vi "TCPClient.vi"() -> ()   [LabVIEW 2020]
uses:
  <vilib>/Analysis/4window.llb/Hanning Window (DBL).vi
  <vilib>/Analysis/4window.llb/AllCosWindow (DBL).vi
  <vilib>/Analysis/NI_AALPro.lvlib
  <vilib>/Analysis/NI_AALBase.lvlib
panel:
  in  "right rank 3":i32=-1
  in  "left rank 3":i32=2
  out "?":i32
  out "max value":i32
  out "Виброускорение":dbl[](graph)
  in  "right rank 2":i32=-1
  in  "left rank 2":i32=2
  in  "right rank":i32=-1
  in  "left rank":i32=2
  out "Виброскорость":dbl[](graph)
  out "Индекс А":i32
  out "Индекс":i32
  out "Максимальная амплитуда на спектре A":dbl
  out "Максимальная амплитуда на спектре S":dbl
  out "error out":errorcluster
  out "Спектр виброускорение":dbl[](graph)
  out "df 2":dbl
  out "СКЗ виброускорения":dbl
  out "Спектр виброскорость":dbl[](graph)
  out "df":dbl
  out "СКЗ Виброскорости":dbl
  out "Виброперемещение":i32[][](graph)
  in  "Connection Uuid":string
  in  "local port (0)":u16
  in  "address 127.0.0.1":string
  # "Панель подключения"
  # "Амплитуда"
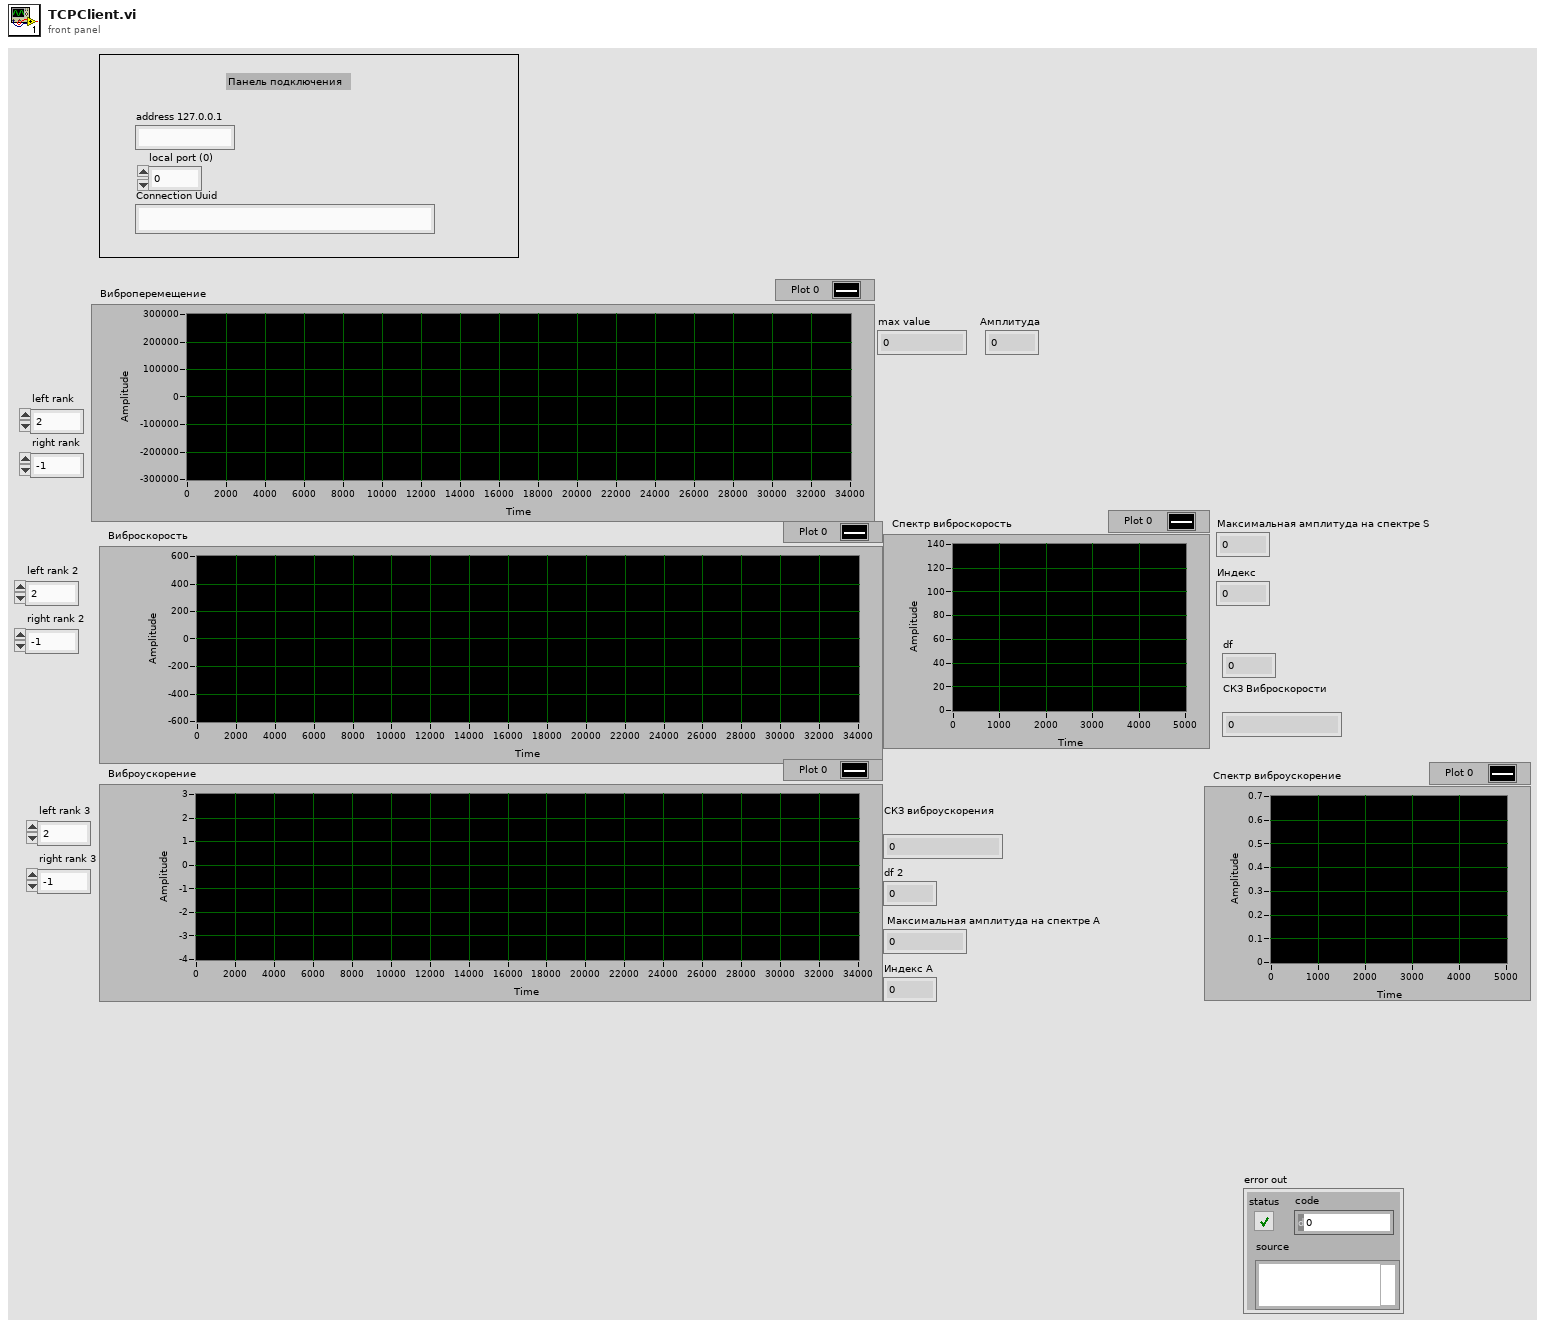
[diagram p1: front panel]
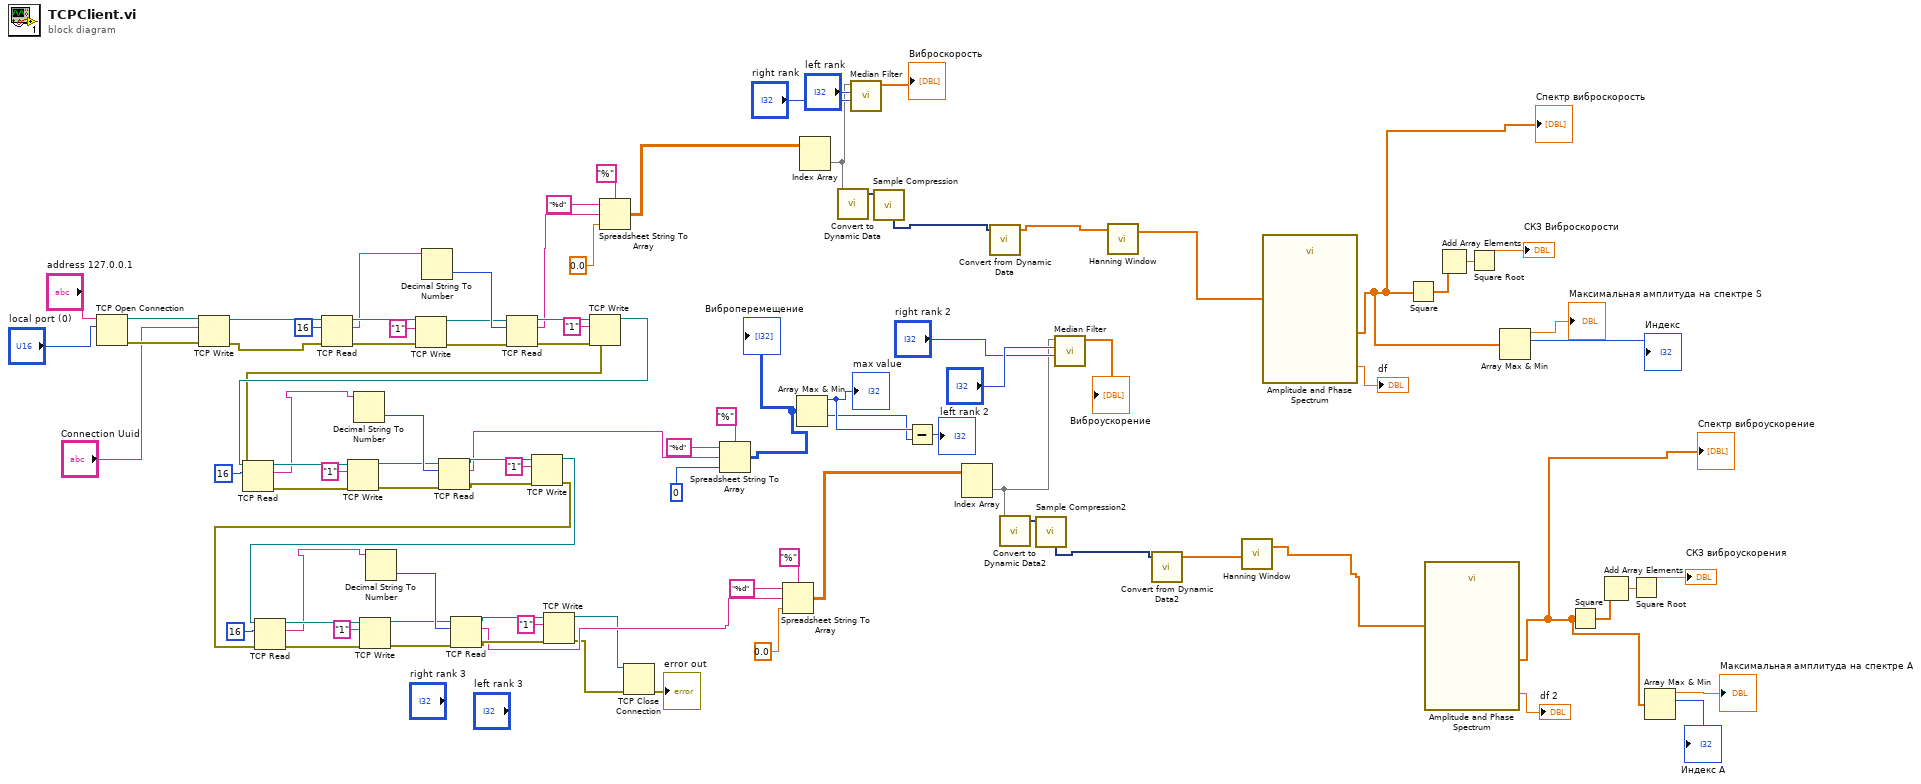
[diagram p0: block diagram]
diagram:
  n1 = TCP Open Connection(address="address 127.0.0.1", remote port or service name="local port (0)") -> (connection ID=w95:refnum<k5>, error out=w94:errorcluster)  [unwired: 3 in]
  n2 = TCP Write(connection ID=w95, data in="Connection Uuid", error in (no error)=w94) -> (connection ID out=w90:refnum<k5>, error out=w91:errorcluster)  [unwired: 1 in, 1 out]
  n3 = TCP Read(connection ID=w90, bytes to read=16, error in (no error)=w91) -> (connection ID out=w87:refnum<k5>, data out=w85:string, error out=w88:errorcluster)  [unwired: 2 in]
  n4 = TCP Write(connection ID=w87, data in="1", error in (no error)=w88) -> (connection ID out=w83:refnum<k5>, error out=w82:errorcluster)  [unwired: 1 in, 1 out]
  n5 = Decimal String To Number(string=w85) -> (number=w84:i32)  [unwired: 2 in, 1 out]
  n6 = TCP Read(connection ID=w83, bytes to read=w84, error in (no error)=w82) -> (connection ID out=w80:refnum<k5>, data out=w17:string, error out=w79:errorcluster)  [unwired: 2 in]
  n7 = TCP Write(connection ID=w80, data in="1", error in (no error)=w79) -> (connection ID out=w53:refnum<k5>, error out=w52:errorcluster)  [unwired: 1 in, 1 out]
  n8 = TCP Read(connection ID=w53, bytes to read=16, error in (no error)=w52) -> (connection ID out=w73:refnum<k5>, data out=w68:string, error out=w74:errorcluster)  [unwired: 2 in]
  n9 = TCP Write(connection ID=w73, data in="1", error in (no error)=w74) -> (connection ID out=w70:refnum<k5>, error out=w69:errorcluster)  [unwired: 1 in, 1 out]
  n10 = Decimal String To Number(string=w68) -> (number=w71:i32)  [unwired: 2 in, 1 out]
  n11 = TCP Read(connection ID=w70, bytes to read=w71, error in (no error)=w69) -> (connection ID out=w65:refnum<k5>, data out=w46:string, error out=w66:errorcluster)  [unwired: 2 in]
  n12 = TCP Write(connection ID=w65, data in="1", error in (no error)=w66) -> (connection ID out=w50:refnum<k5>, error out=w51:errorcluster)  [unwired: 1 in, 1 out]
  n13 = TCP Read(connection ID=w50, bytes to read=16, error in (no error)=w51) -> (connection ID out=w62:refnum<k5>, data out=w57:string, error out=w63:errorcluster)  [unwired: 2 in]
  n14 = TCP Write(connection ID=w62, data in="1", error in (no error)=w63) -> (connection ID out=w59:refnum<k5>, error out=w58:errorcluster)  [unwired: 1 in, 1 out]
  n15 = Decimal String To Number(string=w57) -> (number=w60:i32)  [unwired: 2 in, 1 out]
  n16 = TCP Read(connection ID=w59, bytes to read=w60, error in (no error)=w58) -> (connection ID out=w54:refnum<k5>, data out=w43:string, error out=w55:errorcluster)  [unwired: 2 in]
  n17 = TCP Write(connection ID=w54, data in="1", error in (no error)=w55) -> (connection ID out=w30:refnum<k5>, error out=w29:errorcluster)  [unwired: 1 in, 1 out]
  n18 = Spreadsheet String To Array(delimiter (Tab)="%", format string="%d", spreadsheet string=w17, array type (2D Dbl)=0.0) -> (array=w13:dbl[][])
  n19 = TCP Close Connection(connection ID=w30, error in (no error)=w29) -> (error out=→"error out":errorcluster)  [unwired: 1 in, 1 out]
  n20 = Spreadsheet String To Array(delimiter (Tab)="%", format string="%d", spreadsheet string=w46, array type (2D Dbl)=0) -> (array=w2:i32[][])
  "Виброперемещение" <- w2
  n21 = Spreadsheet String To Array(delimiter (Tab)="%", format string="%d", spreadsheet string=w43, array type (2D Dbl)=0.0) -> (array=w15:dbl[][])
  n22 = Array Max & Min(array=w2) -> (max value=w5:i32, min value=w4:i32)  [unwired: 2 out]
  "max value" <- w5
  n23 = Index Array(array=w13) -> (element=w1:dbl[])  [unwired: 2 in]
  n24 = call "Convert to Dynamic Data"("Array"=w1) -> ("Dynamic Data Type"=w38:dynamicdata)  [unwired: 3 in]
  n25 = call <vilib>:"Median Filter.vi"("right rank"="right rank", "left rank"="left rank", "X"=w1) -> ("Filtered X"=→"Виброскорость":dbl[])  [unwired: 7 in, 1 out]
  n26 = call "Sample Compression"("Signals"=w38) -> ("Last"=w27:dynamicdata)  [unwired: 8 in, 2 out]
  n27 = Subtract(x=w5, y=w4) -> (x-y=→"?":i32)
  n28 = Index Array(array=w15) -> (element=w7:dbl[])  [unwired: 2 in]
  n29 = call "Convert from Dynamic Data"("Dynamic Data Type"=w27) -> ("Array"=w24:dbl[])  [unwired: 3 in]
  n30 = call "Convert to Dynamic Data2"("Array"=w7) -> ("Dynamic Data Type"=w33:dynamicdata)  [unwired: 3 in]
  n31 = call "Sample Compression2"("Signals"=w33) -> ("Last"=w26:dynamicdata)  [unwired: 8 in, 2 out]
  n32 = call <vilib>:"Median Filter.vi"("right rank"="right rank 2", "left rank"="left rank 2", "X"=w7) -> ("Filtered X"=→"Виброускорение":dbl[])  [unwired: 7 in, 1 out]
  n33 = call-poly <vilib>:"Hanning Window.vi"("X"=w24) -> ("Windowed X"=w14:dbl[])  [unwired: 1 out]
  n34 = call "Convert from Dynamic Data2"("Dynamic Data Type"=w26) -> ("Array"=w25:dbl[])  [unwired: 3 in]
  n35 = call-poly <vilib>:"Hanning Window.vi"("X"=w25) -> ("Windowed X"=w16:dbl[])  [unwired: 1 out]
  n36 = call <vilib>:"Amplitude and Phase Spectrum.vi"("Signal (V)"=w14) -> ("df"=→"df":dbl, "Amp Spectrum Mag (Vrms)"=w23:dbl[])  [unwired: 2 in, 1 out]
  "Спектр виброскорость" <- w23
  n37 = Square(x=w23) -> (x^2=w41:dbl[])
  n38 = call <vilib>:"Amplitude and Phase Spectrum.vi"("Signal (V)"=w16) -> ("df"=→"df 2":dbl, "Amp Spectrum Mag (Vrms)"=w21:dbl[])  [unwired: 2 in, 1 out]
  "Спектр виброускорение" <- w21
  n39 = Add Array Elements(numeric array=w41) -> (sum=w40:dbl)
  n40 = Square Root(x=w40) -> (sqrt(x)=→"СКЗ Виброскорости":dbl)
  n41 = Array Max & Min(array=w23) -> (max value=→"Максимальная амплитуда на спектре S":dbl, max index (indices)=→"Индекс":i32)  [unwired: 2 out]
  n42 = Square(x=w21) -> (x^2=w36:dbl[])
  n43 = Add Array Elements(numeric array=w36) -> (sum=w35:dbl)
  n44 = Square Root(x=w35) -> (sqrt(x)=→"СКЗ виброускорения":dbl)
  n45 = Array Max & Min(array=w21) -> (max value=→"Максимальная амплитуда на спектре A":dbl, max index (indices)=→"Индекс А":i32)  [unwired: 2 out]
